vi "WILT Get General Configuration Info.vi"(8 "Error In":errorcluster, 11 "all rows":string[](array[string])) -> (0 "Error Out":errorcluster, 1 "Current Threshold":dbl, 2 "Save Rate":dbl, 3 "Scan Rate":dbl, 4 "Send Restart Every? (Sec)":dbl)   [LabVIEW 2016]
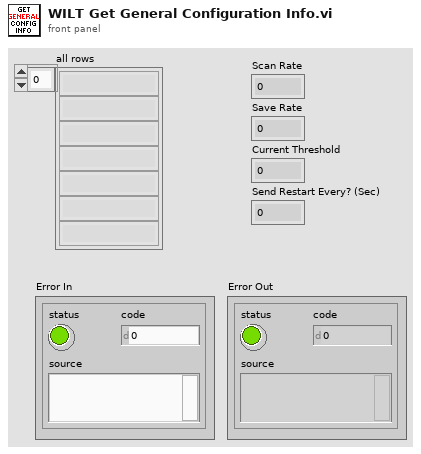
[diagram p1: front panel]
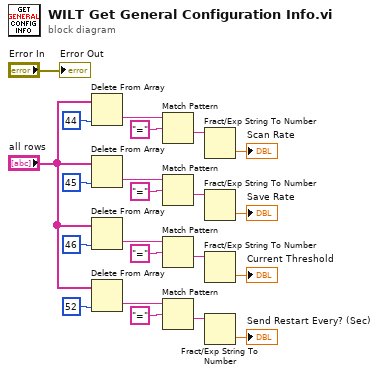
[diagram p0: block diagram]
diagram:
  n1 = Delete From Array(array="all rows", index=44) -> (deleted portion=w6:string)  [unwired: 1 in, 1 out]
  n2 = Delete From Array(array="all rows", index=45) -> (deleted portion=w10:string)  [unwired: 1 in, 1 out]
  n3 = Delete From Array(array="all rows", index=46) -> (deleted portion=w13:string)  [unwired: 1 in, 1 out]
  n4 = Delete From Array(array="all rows", index=52) -> (deleted portion=w16:string)  [unwired: 1 in, 1 out]
  n5 = Match Pattern(string=w6, regular expression="=") -> (after substring=w8:string)  [unwired: 1 in, 3 out]
  n6 = Match Pattern(string=w10, regular expression="=") -> (after substring=w11:string)  [unwired: 1 in, 3 out]
  n7 = Match Pattern(string=w13, regular expression="=") -> (after substring=w14:string)  [unwired: 1 in, 3 out]
  n8 = Match Pattern(string=w16, regular expression="=") -> (after substring=w15:string)  [unwired: 1 in, 3 out]
  n9 = Fract/Exp String To Number(string=w8) -> (number=→"Scan Rate":dbl)  [unwired: 3 in, 1 out]
  n10 = Fract/Exp String To Number(string=w11) -> (number=→"Save Rate":dbl)  [unwired: 3 in, 1 out]
  n11 = Fract/Exp String To Number(string=w14) -> (number=→"Current Threshold":dbl)  [unwired: 3 in, 1 out]
  n12 = Fract/Exp String To Number(string=w15) -> (number=→"Send Restart Every? (Sec)":dbl)  [unwired: 3 in, 1 out]
  "Error Out" <- "Error In"
